vi "ISX3_Example_Measure.vi"() -> ()   [LabVIEW 2012, in "Sciospec ISX3 Impedance Analyzer.lvlib"]
uses:
  Sciospec ISX3 Impedance Analyzer.lvlib
panel:
  out "SpecCount":u16
  out "Current Incoming row":u16
  out "Imag":cluster{dbl[], "Imag":dbl[]}(graph)
  out "Real":cluster{dbl[], "Real":dbl[]}(graph)
  in  "Stopp":bool
  out "ACK for Start CMD":u8[](array[numeric])
  in  "Number of Spectra":u16=1
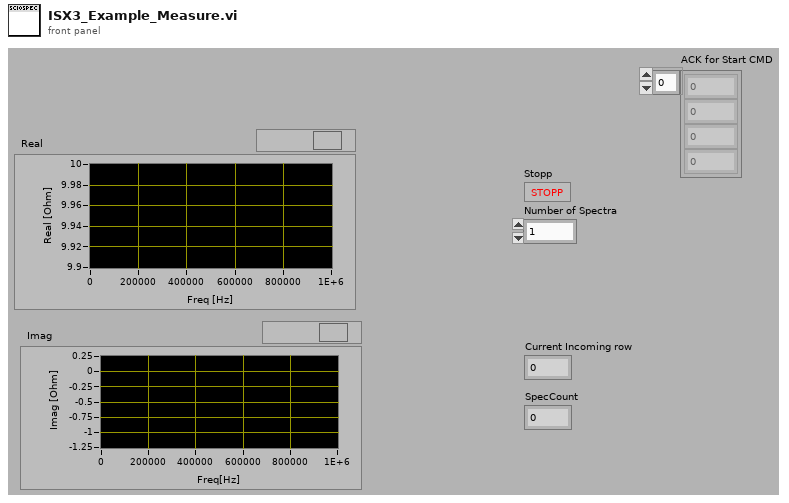
[diagram p1: front panel]
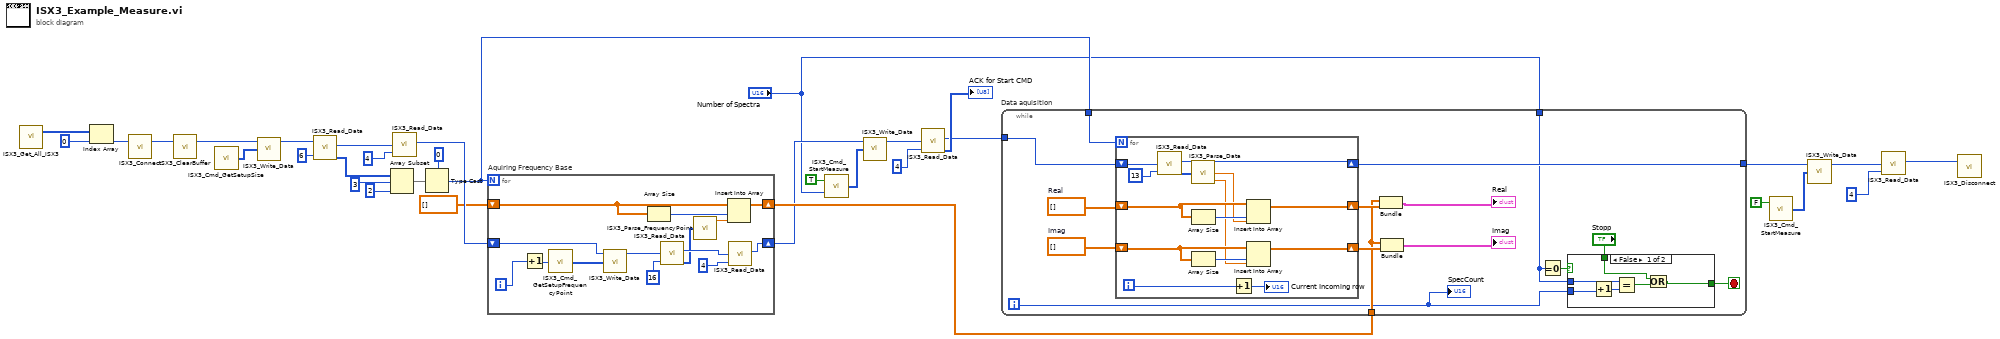
[diagram p0: block diagram]
diagram:
  n1 = call "ISX3_Get_All_ISX3.vi"() -> ("A list of FT_Handel where an ISX-3 is connected to.\nThis handle must be used for further interaction \nwith the USB interface."=w16:u32[])  [unwired: 2 in]
  n2 = Index Array(array=w16, index=u32 0) -> (element=w15:u32)
  n3 = call "ISX3_Connect.vi"("Connect to device with\nFT_Handle"=w15) -> ("Connected to device:"=w2:u32)  [unwired: 2 in]
  n4 = call "ISX3_ClearBuffer.vi"("Handle"=w2) -> ("Handle"=w1:u32)  [unwired: 1 in, 1 out]
  n5 = call "ISX3_Cmd_GetSetupSize.vi"() -> ("get Setup Size Cmd"=w13:u8[])  [unwired: 1 in]
  n6 = call "ISX3_Write_Data.vi"("Data to Write"=w13, "FT_Handle"=w1) -> ("FT_Handle"=w14:u32)  [unwired: 2 in, 1 out]
  n7 = call "ISX3_Read_Data.vi"("FT_Handle"=w14, "Bytes To Read"=6) -> ("Handle"=w27:u32, "Read Data"=w25:u8[])  [unwired: 2 in, 1 out]
  n8 = Array Subset(array=w25, index=3, length=2) -> (w26:u8[])
  n9 = call "ISX3_Read_Data.vi"("FT_Handle"=w27, "Bytes To Read"=4) -> ("Handle"=w21:u32)  [unwired: 2 in, 2 out]
  n10 = Type Cast(type=u16 0, x=w26) -> (*(type *) &x=w18:u16)
  n11 = for "Aquiring Frequency Base" {
    N: w18 -> [_]
    shift-right: [w43] -> w20
    shift-left: dbl[] [] -> [w44]
    shift-right: [w40] -> w12
    shift-left: w21 -> [w38]
    i -> [w47]
    n12 = Increment(x=w47) -> (x+1=w39:i32)
    n13 = call "ISX3_Cmd_GetSetupFrequencyPoint.vi"("Row"=w39) -> ("get Setup Frequency Point Cmd"=w37:u8[])
    n14 = call "ISX3_Write_Data.vi"("Data to Write"=w37, "FT_Handle"=w38) -> ("FT_Handle"=w36:u32)  [unwired: 2 in, 1 out]
    n15 = Array Size(array=w44) -> (size(s)=w45:i32)
    n16 = call "ISX3_Read_Data.vi"("FT_Handle"=w36, "Bytes To Read"=16) -> ("Handle"=w42:u32, "Read Data"=w35:u8[])  [unwired: 2 in, 1 out]
    n17 = call "ISX3_Parse_FrequencyPoint.vi"("Array"=w35) -> ("Frequency [Hz]"=w34:sgl)  [unwired: 2 out]
    n18 = Insert Into Array(array=w44, index=w45, new element=w34) -> (w43:dbl[])
    n19 = call "ISX3_Read_Data.vi"("FT_Handle"=w42, "Bytes To Read"=4) -> ("Handle"=w40:u32)  [unwired: 2 in, 2 out]
  }
  n20 = call "ISX3_Cmd_StartMeasure.vi"("Number of Spectra"="Number of Spectra", "Start/Stop"=TRUE) -> ("Start/Stop measurement cmd"=w8:u8[])
  n21 = call "ISX3_Write_Data.vi"("Data to Write"=w8, "FT_Handle"=w12) -> ("FT_Handle"=w11:u32)  [unwired: 2 in, 1 out]
  n22 = call "ISX3_Read_Data.vi"("FT_Handle"=w11, "Bytes To Read"=4) -> ("Handle"=w30:u32, "Read Data"=→"ACK for Start CMD":u8[])  [unwired: 2 in, 1 out]
  n23 = while "Data aquisition" {
    tunnel: w30 -> [w62]
    tunnel: [w59] -> w5
    tunnel: w20 -> [w56]
    tunnel: "Number of Spectra" -> [w52]
    tunnel: w18 -> [w48]
    i -> [w49]
    stop <- w51 stop-if-true
    w60 = dbl[] []  # Imag
    w61 = dbl[] []  # Real
    n24 = for {
      N: w48 -> [_]
      shift-right: [w82] -> w59
      shift-left: w62 -> [w83]
      shift-right: [w77] -> w58
      shift-left: w61 -> [w75]
      shift-right: [w79] -> w57
      shift-left: w60 -> [w80]
      i -> [w74]
      n25 = call "ISX3_Read_Data.vi"("FT_Handle"=w83, "Bytes To Read"=13) -> ("Handle"=w82:u32, "Read Data"=w70:u8[])  [unwired: 2 in, 1 out]
      n26 = call "ISX3_Parse_Data.vi"("Array"=w70) -> ("Real"=w72:sgl, "Imag"=w71:sgl)  [unwired: 1 out]
      n27 = Array Size(array=w75) -> (size(s)=w78:i32)
      n28 = Array Size(array=w80) -> (size(s)=w81:i32)
      n29 = Increment(x=w74) -> (x+1=→"Current Incoming row":i32)
      n30 = Insert Into Array(array=w75, index=w78, new element=w72) -> (w77:dbl[])
      n31 = Insert Into Array(array=w80, index=w81, new element=w71) -> (w79:dbl[])
    }
    n32 = Bundle(w56, "Real"=w58) -> (→"Real":cluster{dbl[], "Real":dbl[]})  [unwired: 1 in]
    n33 = Bundle(w56, "Imag"=w57) -> (→"Imag":cluster{dbl[], "Imag":dbl[]})  [unwired: 1 in]
    n34 = Equal To 0?(x=w52) -> (x = 0?=w53:bool)
    n35 = case shown="False" w53 {
      tunnel: w52 -> [w68 _]
      tunnel: w49 -> [w67 _]
      tunnel: [w65 w69] -> w51
      tunnel: "Stopp" -> [w64 w69]
      frame False {
        n36 = Increment(x=w67) -> (x+1=w66:i32)
        n37 = Equal?(x=w68, y=w66) -> (x = y?=w63:bool)
        n38 = Or(x=w64, y=w63) -> (x .or. y?=w65:bool)
      }
      frame True {
      }
    }
    "SpecCount" <- w49
  }
  n39 = call "ISX3_Cmd_StartMeasure.vi"("Start/Stop"=FALSE) -> ("Start/Stop measurement cmd"=w6:u8[])  [unwired: 1 in]
  n40 = call "ISX3_Write_Data.vi"("Data to Write"=w6, "FT_Handle"=w5) -> ("FT_Handle"=w4:u32)  [unwired: 2 in, 1 out]
  n41 = call "ISX3_Read_Data.vi"("FT_Handle"=w4, "Bytes To Read"=4) -> ("Handle"=w3:u32)  [unwired: 2 in, 2 out]
  n42 = call "ISX3_Disconnect.vi"("FT_Handle"=w3) -> ()  [unwired: 2 in]
